vi "英维克空调.vi"() -> ()   [LabVIEW 2016, in "环境动力监测库.lvlib" / "空调库.lvlib"]
uses:
  <vilib>/Utility/config.llb/NI_LVConfig.lvlib
  <vilib>/ptbypt/NI_PtbyPt.lvlib
panel:
  out "遥控开关机状态":bool
  in  "重开串口":bool
  in  "设定参数":bool
  in  "遥控":bool
  out "系统参数":T1
  out "告警状态":T2
  out "传感器状态":T3
  out "运行状态":T4
  out "通讯":bool
  out "VISA resource name":refnum<visa-resource-name>="COM10" caption="VISA资源名称"
  # "英维克空调"
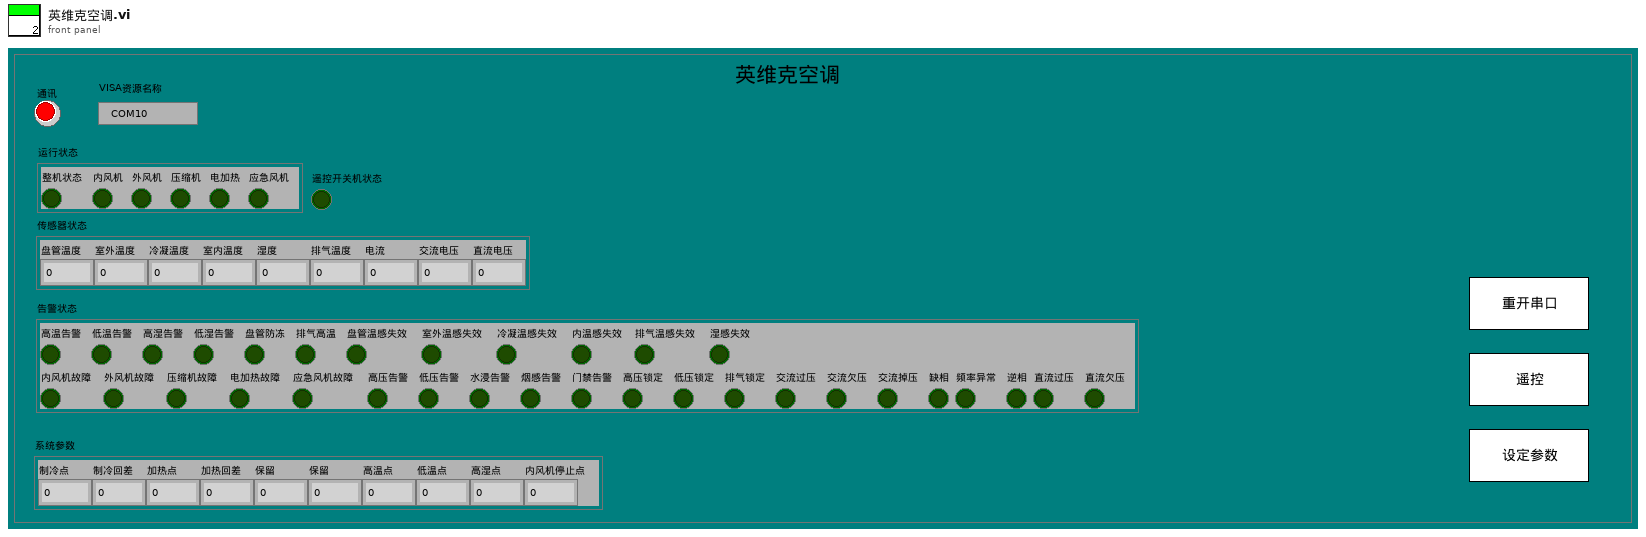
[diagram p1: front panel]
types:
  T1 = cluster{"制冷点":u16, "制冷回差":u16, "加热点":u16, "加热回差":u16, "保留":u16, "保留":u16, "高温点":u16, "低温点":u16, "高湿点":u16, "内风机停止点":u16}
  T2 = cluster{"高温告警":bool, "低温告警":bool, "高湿告警":bool, "低湿告警":bool, "盘管防冻":bool, "排气高温":bool, "盘管温感失效":bool, "室外温感失效":bool, "冷凝温感失效":bool, "内温感失效":bool, "排气温感失效":bool, "湿感失效":bool, "内风机故障":bool, "外风机故障":bool, "压缩机故障":bool, "电加热故障":bool, "应急风机故障":bool, "高压告警":bool, "低压告警":bool, "水浸告警":bool, "烟感告警":bool, "门禁告警":bool, "高压锁定":bool, "低压锁定":bool, "排气锁定":bool, "交流过压":bool, "交流欠压":bool, "交流掉压":bool, "缺相":bool, "频率异常":bool, "逆相":bool, "直流过压":bool, "直流欠压":bool}
  T3 = cluster{"盘管温度":u16, "室外温度":u16, "冷凝温度":u16, "室内温度":u16, "湿度":u16, "排气温度":u16, "电流":u16, "交流电压":u16, "直流电压":u16}
  T4 = cluster{"整机状态":bool, "内风机":bool, "外风机":bool, "压缩机":bool, "电加热":bool, "应急风机":bool}
  T5 = typedef "NI_LVConfig.lvlib/Config Data RefNum.ctl" = refnum<k1>
  T6 = cluster{"漏水监测输出":bool, "门禁监测输出":bool, "温湿度监测输出":bool, "烟雾监测输出":bool, "空调监测输出":bool, "自动重合闸输出":bool}
  T7 = enum16{"空调制冷点", "空调制冷回差", "加热点", "加热回差", "高温点", "低温点", "高湿点", "内风机停止点"}
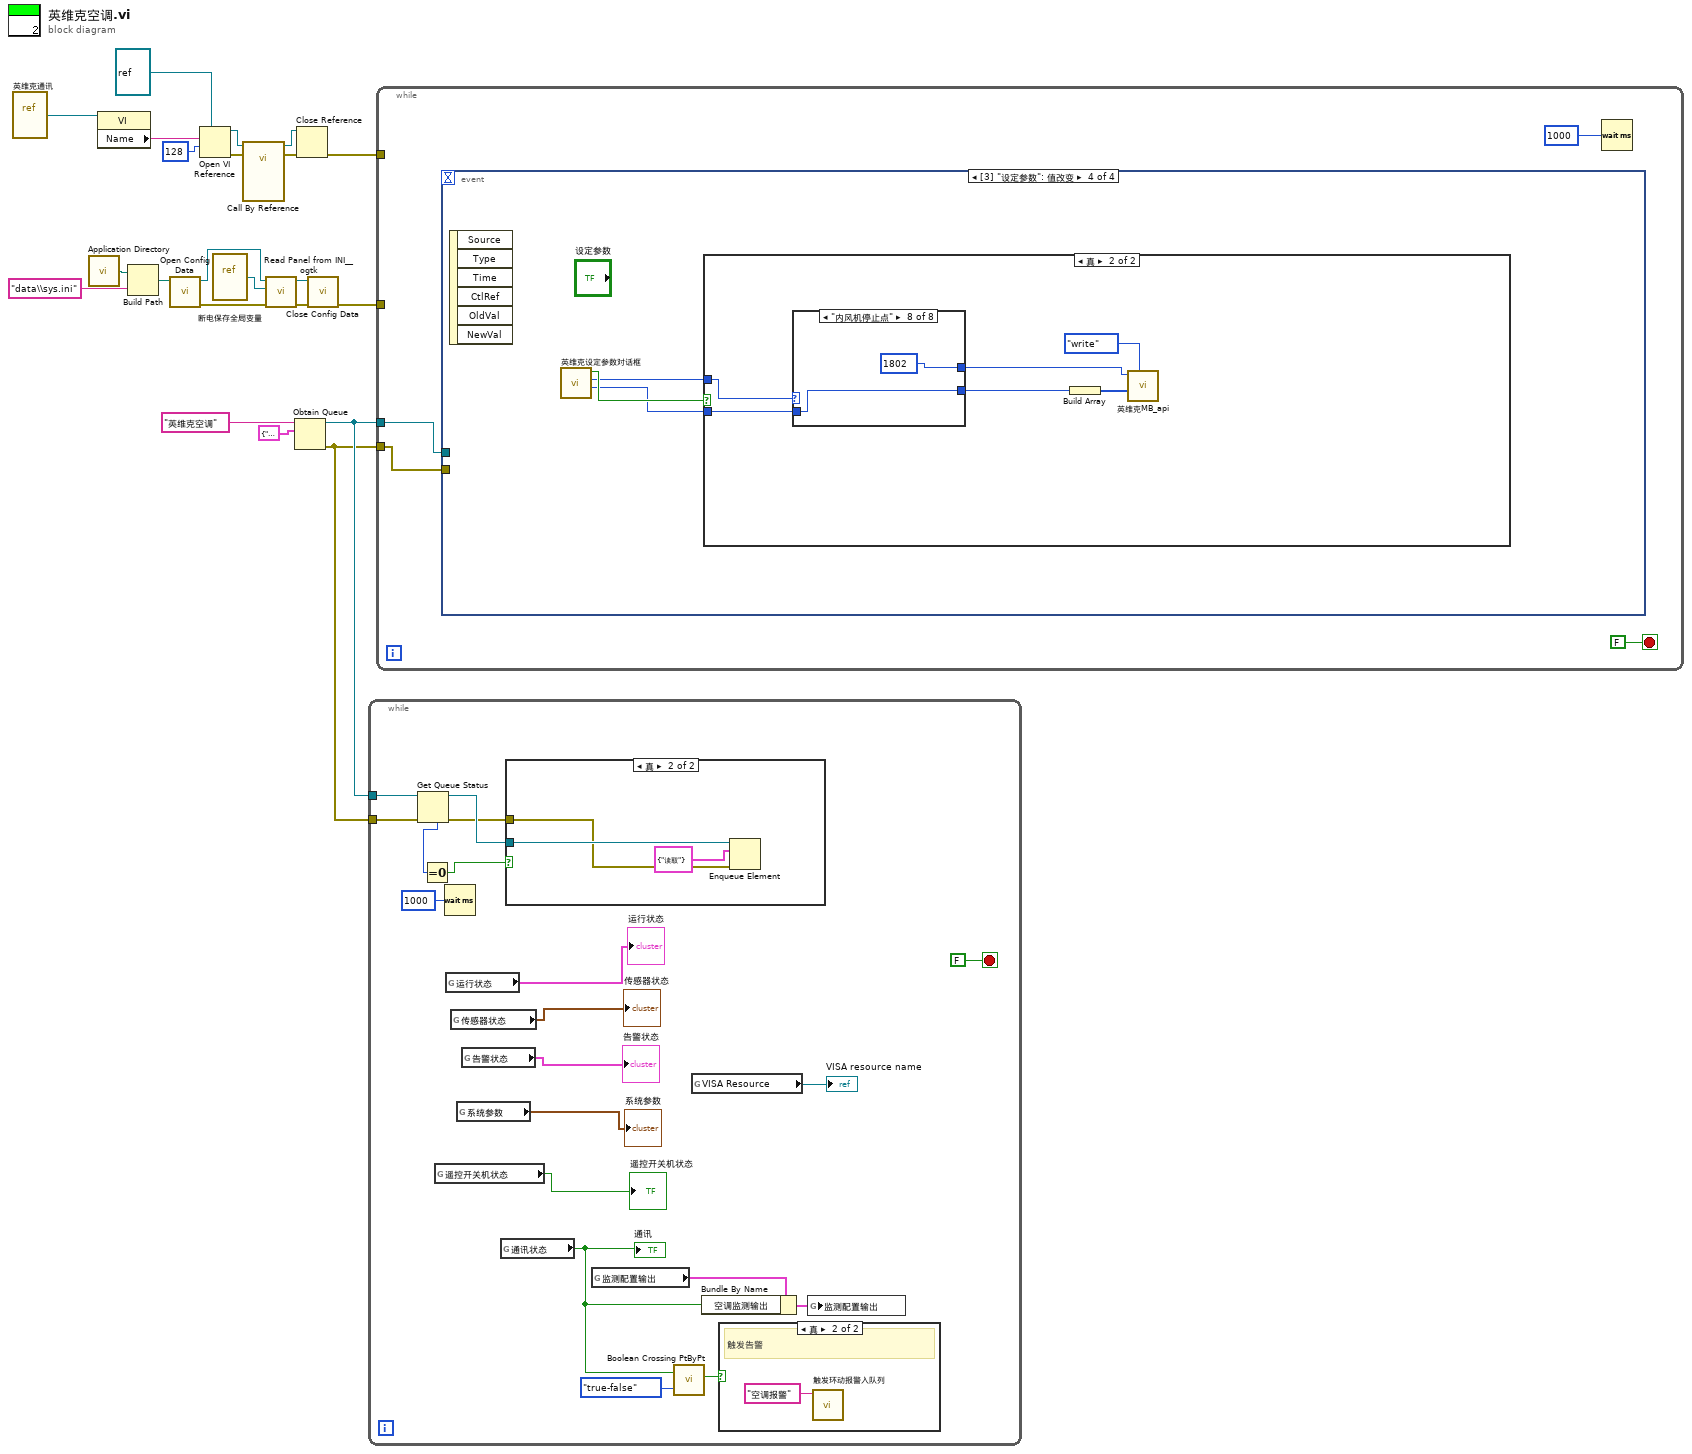
[diagram p0: block diagram]
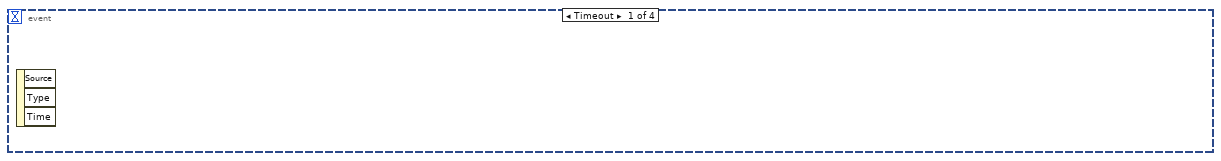
[diagram p4: hidden frame]
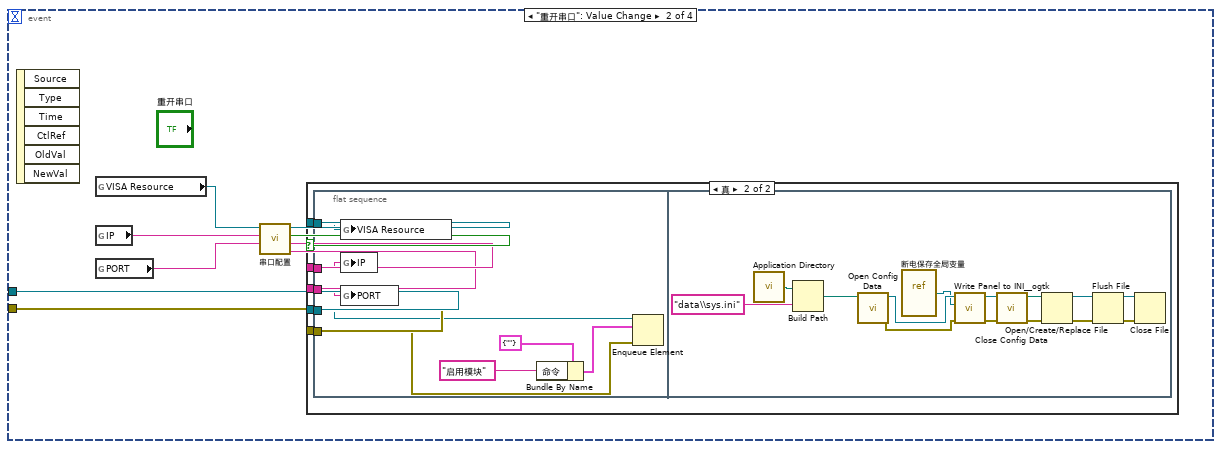
[diagram p5: hidden frame]
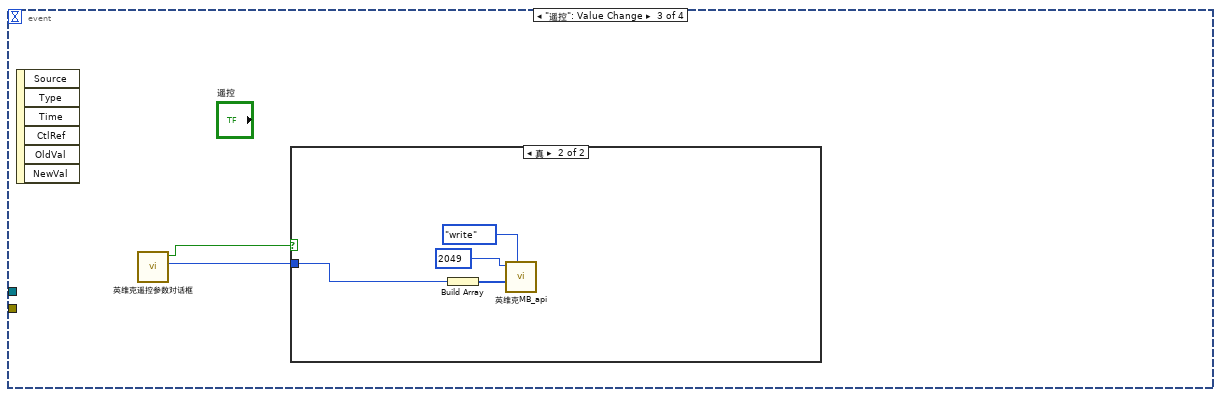
[diagram p7: hidden frame]
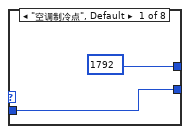
[diagram p10: hidden frame]
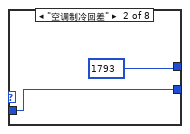
[diagram p11: hidden frame]
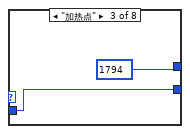
[diagram p12: hidden frame]
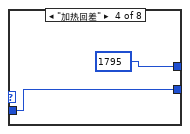
[diagram p13: hidden frame]
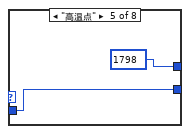
[diagram p14: hidden frame]
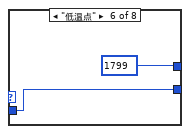
[diagram p15: hidden frame]
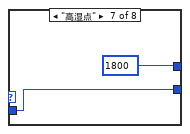
[diagram p16: hidden frame]
diagram:
  n1 = vi-ref "英维克通讯.vi"() -> (w15:refnum<vi>)
  n2 = call <vilib>:"Application Directory.vi"() -> ("Application Directory"=w13:path)
  n3 = property class="VI"(reference=w15) -> ("Name"=w16:string)  [unwired: 1 in, 2 out]
  n4 = Build Path(base path=w13, name or relative path="data\\sys.ini" ("名称或相对路径")) -> (appended path=w11:path)
  n5 = call <vilib>:"Open Config Data.vi"("configuration file path"=w11) -> ("error out"=w7:errorcluster, "refnum"=w10:T5)  [unwired: 8 in, 1 out]
  n6 = Open VI Reference(type specifier VI Refnum (for type only)=refnum<vi> refnum, vi path=w16, options=128 ("选项")) -> (vi reference=w18:refnum<vi>, error out=w20:errorcluster)  [unwired: 3 in]
  n7 = vi-ref "断电保存全局变量.vi"() -> (w9:refnum<vi>)
  n8 = call-by-ref "?"(reference=w18, error in=w20) -> (reference out=w22:refnum<vi>, error out=w21:errorcluster)  [unwired: 12 in]
  n9 = call <userlib>:"Read Panel from INI__ogtk.vi"("error in (no error)"=w7, "VI ref"=w9, "refnum"=w10) -> ("error out"=w6:errorcluster, "refnum out"=w8:T5)  [unwired: 7 in]
  n10 = Obtain Queue(name (unnamed)="英维克空调" ("名称（未命名）"), element data type=cluster{"命令":string} {"命令"="启用模块"} ("元素")) -> (queue out=w2:refnum<queue>, error out=w1:errorcluster)  [unwired: 3 in, 1 out]
  n11 = Close Reference(reference=w22, error in (no error)=w21) -> (error out=w14:errorcluster)
  n12 = call <vilib>:"Close Config Data.vi"("error in (no error)"=w6, "refnum"=w8) -> ("error out"=w5:errorcluster)  [unwired: 8 in, 1 out]
  n13 = while {
    tunnel: w2 -> [w40]
    tunnel: w1 -> [w39]
    stop <- FALSE stop-if-true
    n14 = Get Queue Status(queue=w40, error in (no error)=w39) -> (queue out=w37:refnum<queue>, error out=w36:errorcluster, # elements in queue=w41:i32)  [unwired: 1 in, 5 out]
    n15 = Equal To 0?(x=w41) -> (x = 0?=w38:bool)
    n16 = global read "内部交互全局变量.vi" "遥控开关机状态"() -> (→"遥控开关机状态":bool)
    n17 = Wait (ms)(milliseconds to wait=u32 1000 ("等待时间（毫秒）")) -> ()  [unwired: 1 out]
    n18 = global read "内部交互全局变量.vi" "运行状态"() -> (→"运行状态":T4)
    n19 = global read "内部交互全局变量.vi" "传感器状态"() -> (→"传感器状态":T3)
    n20 = global read "内部交互全局变量.vi" "系统参数"() -> (→"系统参数":T1)
    n21 = global read "内部交互全局变量.vi" "告警状态"() -> (→"告警状态":T2)
    n22 = global read "断电保存全局变量.vi" "通讯状态"() -> (w23:bool)
    "通讯" <- w23
    n23 = case shown="真" w38 {
      tunnel: w37 -> [_ w45]
      tunnel: w36 -> [_ w44]
      frame False {
      }
      frame True {
        n24 = Enqueue Element(queue=w45, element=cluster{"命令":string} {"命令"="读取"} ("元素"), error in (no error)=w44) -> ()  [unwired: 1 in, 3 out]
      }
    }
    n25 = global read "内部交互全局变量.vi" "监测配置输出"() -> (w27:T6)
    n26 = call <vilib>:"Boolean Crossing PtByPt.vi"("direction"=enum16{"either", "false-true", "true-false"}."true-false", "input"=w23) -> ("crossing"=w24:bool)  [unwired: 1 in]
    n27 = global read "断电保存全局变量.vi" "VISA Resource"() -> (→"VISA resource name":refnum<visa-resource-name>)
    n28 = Bundle By Name(cluster=w27, "空调监测输出"=w23) -> (w26:T6)
    n29 = case shown="真" w24 {
      frame False {
      }
      frame True {
        # "触发告警"
        n30 = call "触发环动报警入队列.vi"("报警内容"="空调报警") -> ()  [unwired: 11 in]
      }
    }
    n31 = global write "内部交互全局变量.vi" "监测配置输出"(w26) -> ()
  }
  n32 = while {
    tunnel: w14 -> [_]
    tunnel: w5 -> [_]
    tunnel: w2 -> [w47]
    tunnel: w1 -> [w46]
    stop <- FALSE stop-if-true
    n33 = event shown="[3] \"设定参数\": 值改变" {
      selector: _ -> [_ _ _ _]
      dyn-events: _ -> [_ _ _ _]
      timeout: _ -> [_ _ _ _]
      tunnel: w47 -> [_ w51 _ _]
      tunnel: w46 -> [_ w50 _ _]
      event Timeout {
        n34 = event-data() -> ()  [unwired: 1 in, 3 out]
      }
      event "重开串口": Value Change {
        n35 = event-data() -> ()  [unwired: 1 in, 6 out]
        n36 = global read "断电保存全局变量.vi" "VISA Resource"() -> (w58:refnum<visa-resource-name>)
        n37 = global read "断电保存全局变量.vi" "IP"() -> (w53:string)
        n38 = global read "断电保存全局变量.vi" "PORT"() -> (w52:string)
        n39 = call "串口配置.vi"("PORT"=w52, "IP"=w53, "请选择串口:"=w58) -> ("PORT 2"=w54:string, "IP 2"=w55:string, "确认 2"=w56:bool, "VISA资源名称 2"=w57:refnum<visa-resource-name>)  [unwired: 5 in]
        n40 = case shown="真" w56 {
          tunnel: w57 -> [_ w61]
          tunnel: w51 -> [_ w63]
          tunnel: w50 -> [_ w62]
          tunnel: w55 -> [_ w60]
          tunnel: w54 -> [_ w59]
          frame False {
          }
          frame True {
            n41 = flat-sequence {
              tunnel: w63 -> [w68]
              tunnel: w62 -> [w67]
              tunnel: w61 -> [w66]
              tunnel: w60 -> [w65]
              tunnel: w59 -> [w64]
              frame #0 {
                n42 = global write "断电保存全局变量.vi" "VISA Resource"(w66) -> ()
                n43 = global write "断电保存全局变量.vi" "IP"(w65) -> ()
                n44 = global write "断电保存全局变量.vi" "PORT"(w64) -> ()
                n45 = Bundle By Name(cluster=cluster{"命令":string} {"命令"=""} ("元素"), "命令"="启用模块" ("名称（未命名）")) -> (w69:cluster{"命令":string})
                n46 = Enqueue Element(queue=w68, element=w69, error in (no error)=w67) -> ()  [unwired: 1 in, 3 out]
              }
              frame #1 {
                n47 = call <vilib>:"Application Directory.vi"() -> ("Application Directory"=w84:path)
                n48 = Build Path(base path=w84, name or relative path="data\\sys.ini" ("名称或相对路径")) -> (appended path=w83:path)
                n49 = call <vilib>:"Open Config Data.vi"("configuration file path"=w83) -> ("error out"=w79:errorcluster, "refnum"=w82:T5)  [unwired: 8 in, 1 out]
                n50 = vi-ref "断电保存全局变量.vi"() -> (w81:refnum<vi>)
                n51 = call <userlib>:"Write Panel to INI__ogtk.vi"("error in (no error)"=w79, "VI ref"=w81, "refnum"=w82) -> ("error out"=w78:errorcluster, "refnum out"=w80:T5)  [unwired: 7 in]
                n52 = call <vilib>:"Close Config Data.vi"("error in (no error)"=w78, "refnum"=w80) -> ("error out"=w73:errorcluster, "file path"=w72:path)  [unwired: 8 in]
                n53 = Open/Create/Replace File(file path (use dialog)=w72, error in=w73) -> (refnum out=w76:refnum<file>, error out=w77:errorcluster)  [unwired: 4 in, 1 out]
                n54 = Flush File(refnum=w76, error in=w77) -> (refnum out=w75:refnum<file>, error out=w74:errorcluster)
                n55 = Close File(refnum=w75, error in=w74) -> ()  [unwired: 2 out]
              }
            }
          }
        }
      }
      event "遥控": Value Change {
        n56 = event-data() -> ()  [unwired: 1 in, 6 out]
        n57 = call "英维克遥控参数对话框.vi"() -> ("遥控参数选择输出"=w86:enum16{"空调关机", "空调开机"}, "确定?"=w87:bool)  [unwired: 10 in]
        n58 = case shown="真" w87 {
          tunnel: w86 -> [_ w89]
          frame False {
          }
          frame True {
            n59 = Build Array(w89) -> (w88:enum16{"空调关机", "空调开机"}[])
            n60 = call "英维克MB_api.vi"("STEP"=enum16{"open", "read", "write", "close"}."write", "values"=w88, "starting address"=u16 2049) -> ()  [unwired: 6 in, 3 out]
          }
        }
      }
      event "设定参数": Value Change {
        n61 = event-data() -> ()  [unwired: 1 in, 6 out]
        n62 = call "英维克设定参数对话框.vi"() -> ("参数 2"=w92:u16, "设定参数（定点数）选择 2"=w93:T7, "确定?"=w94:bool)  [unwired: 9 in]
        n63 = case shown="真" w94 {
          tunnel: w93 -> [_ w100]
          tunnel: w92 -> [_ w96]
          frame False {
          }
          frame True {
            n64 = case shown="\"内风机停止点\"" w100 {
              tunnel: [u16 1792 ("starting address") u16 1793 ("starting address") u16 1794 ("starting address") u16 1795 ("starting address") u16 1798 ("starting address") u16 1799 ("starting address") u16 1800 ("starting address") u16 1802 ("starting address")] -> w97
              tunnel: w96 -> [w101 w103 w105 w107 w109 w111 w113 w115]
              tunnel: [w101 w103 w105 w107 w109 w111 w113 w115] -> w95
              frame "空调制冷点", Default {
              }
              frame "空调制冷回差" {
              }
              frame "加热点" {
              }
              frame "加热回差" {
              }
              frame "高温点" {
              }
              frame "低温点" {
              }
              frame "高湿点" {
              }
              frame "内风机停止点" {
              }
            }
            n65 = Build Array(w95) -> (w98:u16[])
            n66 = call "英维克MB_api.vi"("STEP"=enum16{"open", "read", "write", "close"}."write", "values"=w98, "starting address"=w97) -> ()  [unwired: 6 in, 3 out]
          }
        }
      }
    }
    n67 = Wait (ms)(milliseconds to wait=u32 1000 ("等待时间（毫秒）")) -> ()  [unwired: 1 out]
  }
